vi "_xxxxx.vi"() -> (2 "Msg Strategy":refnum<class "Msg Strategy.lvclass">)   [LabVIEW 2021, in "Providers.lvlib" / "jettl Msg xxxxx.lvlib"]
uses:
  jettl Msg xxxxx.lvlib
  jettl/Msg Strategy/Msg Strategy.lvclass
  xxxxx Msg Strategy/xxxxx Msg Strategy.lvclass
  C:/git/jettl/src/jettl/Msg Strategy/Msg Strategy.lvclass
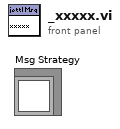
[diagram p1: front panel]
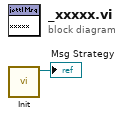
[diagram p0: block diagram]
diagram:
  n1 = call "Init.vi"() -> ("xxxxx Msg Strategy out"=→"Msg Strategy":refnum<class "xxxxx Msg Strategy.lvclass">)  [unwired: 11 in]
